vi "Next Step.vi"(8 "error in (no error)":errorcluster, 11 "Magnetic Field Lakeshore Continuous in":refnum<class "Magnetic Field Lakeshore Continuous.lvclass">) -> (0 "error out":errorcluster, 1 "Current Step":u32, 2 "actual position":dbl, 3 "Magnetic Field Lakeshore Continuous out":refnum<class "Magnetic Field Lakeshore Continuous.lvclass">)   [LabVIEW 2023, in "Magnetic Field Lakeshore Continuous.lvclass"]
doc: "(Dynamic) Move to the next preconfigured step of this Scanner, and return the current position (actual, not intended) of this Scanner. Increment the step counter by one."
uses:
  Magnetic Field Lakeshore Continuous.lvclass
  Scanner/Scanner.lvclass
  Instruments/Utility Classes/Scannable/Scannable.lvclass
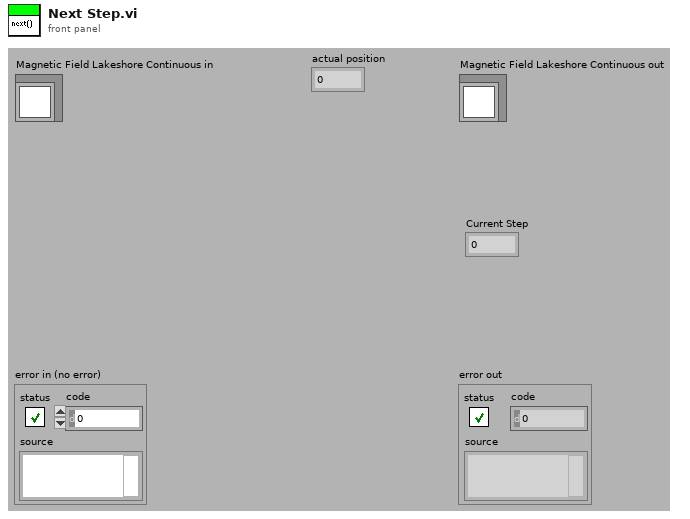
[diagram p1: front panel]
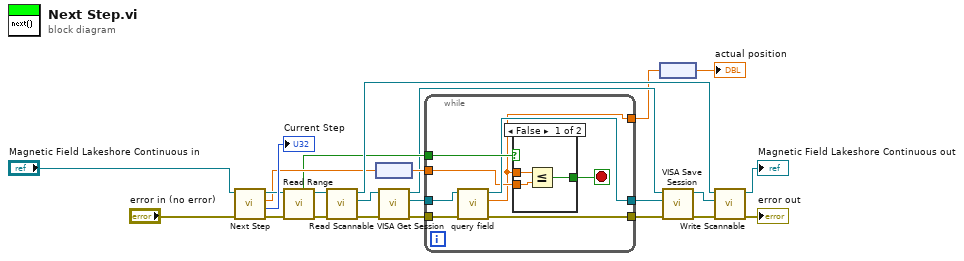
[diagram p0: block diagram]
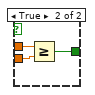
[diagram p2: hidden frame]
diagram:
  n1 = call-parent "Next Step.vi"("error in (no error)"="error in (no error)", "Scanner in"="Magnetic Field Lakeshore Continuous in") -> ("error out"=w21:errorcluster, "Current Step"=→"Current Step":u32, "Current Position"=w6:dbl, "Scanner out"=w14:refnum<class "Magnetic Field Lakeshore Continuous.lvclass">)  [unwired: 6 in]
  n2 = call-dynamic "Read Range.vi"("error in (no error)"=w21, "Scanner.lvclass in"=w14) -> ("error out"=w20:errorcluster, "Scanner.lvclass out"=w13:refnum<class "Magnetic Field Lakeshore Continuous.lvclass">, "Scanning Up?"=w4:bool)  [unwired: 7 out]
  n3 = call-dynamic "Read Scannable.vi"("error in (no error)"=w20, "Scanner.lvclass in"=w13) -> ("error out"=w19:errorcluster, "Scannable.lvclass"=w10:refnum<class "Scannable.lvclass">, "Scanner.lvclass out"=w12:refnum<class "Magnetic Field Lakeshore Continuous.lvclass">)  [unwired: 7 in]
  n4 = node(w6) -> (w5:dbl[unit])
  n5 = call-dynamic "VISA Get Session.vi"("error in (no error)"=w19, "Instrument.lvclass in"=w10) -> ("error out"=w17:errorcluster, "VISA Resource Name"=w8:refnum<visa-resource-name>, "Instrument.lvclass out"=w3:refnum<class "Scannable.lvclass">)  [unwired: 7 out]
  n6 = while {
    tunnel: [w28] -> w18
    tunnel: w17 -> [w29]
    tunnel: w8 -> [w31]
    tunnel: [w30] -> w7
    tunnel: w5 -> [w27]
    tunnel: w4 -> [w32]
    tunnel: [w25] -> w2
    stop <- w26 stop-if-true
    n7 = call "query field.vi"("error in (no error)"=w29, "VISA session"=w31) -> ("error out"=w28:errorcluster, "Field reading"=w25:dbl[unit], "dup VISA session"=w30:refnum<visa-resource-name>)  [unwired: 7 in]
    n8 = case shown="False" w32 {
      tunnel: w25 -> [w34 w38]
      tunnel: w27 -> [w35 w37]
      tunnel: [w33 w36] -> w26
      frame False {
        n9 = Less Or Equal?(x=w34, y=w35) -> (x <= y?=w33:bool)
      }
      frame True {
        n10 = Greater Or Equal?(x=w38, y=w37) -> (x >= y?=w36:bool)
      }
    }
  }
  n11 = node(w2) -> (→"actual position":dbl)
  n12 = call-dynamic "VISA Save Session.vi"("error in (no error)"=w18, "VISA Resource Name"=w7, "Instrument.lvclass in"=w3) -> ("error out"=w16:errorcluster, "Instrument.lvclass out"=w9:refnum<class "Scannable.lvclass">)  [unwired: 7 out]
  n13 = call-dynamic "Write Scannable.vi"("error in (no error)"=w16, "Scannable.lvclass"=w9, "Scanner.lvclass in"=w12) -> ("error out"=→"error out":errorcluster, "Scanner.lvclass out"=→"Magnetic Field Lakeshore Continuous out":refnum<class "Magnetic Field Lakeshore Continuous.lvclass">)  [unwired: 7 in]
